vi "Lab Panel V5.22.vi"() -> ()   [LabVIEW 2013] (continued)
                                n836 = local write "DISP LAB03-2"(w1475) -> ()
                              }
                              frame #4 {
                                n837 = local read "TEMP START LAB03-2"() -> (w1494:cluster{"TL":dbl, "TN":dbl})
                                n838 = Bundle(cluster=w1494, "TL"=w1492, "TN"=w1492) -> (w1493:cluster{"TL":dbl, "TN":dbl})
                                n839 = local write "TEMP START LAB03-2"(w1493) -> ()
                              }
                            }
                          }
                        }
                      }
                    }
                  }
                }
              }
              event "RUN LAB04-1": Value Change {
                n840 = event-data() -> ("NewVal"=w1499:bool)  [unwired: 1 in, 5 out]
                n841 = local write "run lab04-1"(w1499) -> ()
                n842 = case shown="True" w1499 {
                  tunnel: w1505 -> [_ w1543]
                  tunnel: w1504 -> [_ w1542]
                  tunnel: w1502 -> [w1507 w1541]
                  tunnel: w1503 -> [_ w1540]
                  tunnel: w1501 -> [_ w1539]
                  tunnel: [w1506 w1538] -> w1500
                  tunnel: w1498 -> [_ w1537]
                  tunnel: w1497 -> [_ w1536]
                  tunnel: w1496 -> [_ w1535]
                  tunnel: w1495 -> [_ w1533]
                  frame False {
                    # "stop test"
                    n843 = stacked-sequence {
                      tunnel: w1507 -> [w1516 _]
                      tunnel: [w1508 _] -> w1506
                      frame #0 {
                        n844 = local read "DISP LAB04-1"() -> (w1515:T4)
                        n845 = Unbundle(w1515) -> ("CYCLE"=w1513:dbl, "MINS"=w1514:dbl)  [unwired: 1 out]
                        n846 = case shown="\"CYCLE TEST\"" w1516 {
                          tunnel: w1514 -> [_ _ w1523]
                          tunnel: w1513 -> [w1521 w1522 _]
                          tunnel: [w1521 w1522 w1523] -> w1512
                          frame "CHART TEST", Default {
                          }
                          frame "CYCLE TEST" {
                          }
                          frame "T-RISE TEST" {
                          }
                        }
                        n847 = local read "TDMS LAB04-1"() -> (w1520:refnum<k34>)
                        n848 = Build Array("STOPPED") -> (w1517:string[])
                        n849 = Build Array(w1512) -> (w1511:dbl[])
                        n850 = TDMS Write(0:w1520, 5:"TEST RESULT", 7:w1517, 9:w1511) -> (4:w1509:refnum<k34>, 15:w1510:errorcluster)  [unwired: 2 in, 2 out]
                        n851 = TDMS Close(8:w1510, 11:w1509) -> (0:w1508:errorcluster)  [unwired: 1 out]
                      }
                      frame #1 {
                        n852 = local read "DISP LAB04-1"() -> (w1527:T4)
                        n853 = stacked-sequence {
                          tunnel: "LAB04-1" -> [w1529 w1531]
                          frame #0 {
                            n854 = call "sub vi - defrag tdms v1.vi"("panel id"=w1529) -> ("error out"=w1528:errorcluster)  [unwired: 10 in]
                            n855 = local write "data file error"(w1528) -> ()
                          }
                          frame #1 {
                            n856 = call "Save data file (stop) v3.vi"("panel id"=w1531) -> ("network file save error"=w1530:errorcluster)  [unwired: 9 in, 1 out]
                            n857 = local write "RESULT LAB04-1"(FALSE) -> ()
                            n858 = local write "data file error"(w1530) -> ()
                          }
                        }
                        n859 = Bundle(cluster=w1527, "STATUS"="STOP") -> (w1525:T4)  [unwired: 2 in]
                        n860 = local write "DISP LAB04-1"(w1525) -> ()
                      }
                    }
                  }
                  frame True {
                    n861 = local read "SIG LAB04-1"() -> (w1534:T2)
                    n862 = stacked-sequence {
                      seq-local: [w1545 _] -> [_ w1549]
                      tunnel: w1543 -> [_ w1559]
                      tunnel: w1542 -> [_ w1558]
                      tunnel: w1541 -> [_ w1557]
                      tunnel: w1540 -> [_ w1556]
                      tunnel: w1539 -> [_ w1555]
                      tunnel: [_ w1554] -> w1538
                      tunnel: w1537 -> [_ w1553]
                      tunnel: w1536 -> [_ w1552]
                      tunnel: w1535 -> [_ w1551]
                      tunnel: w1534 -> [w1544 w1550]
                      tunnel: w1533 -> [_ w1548]
                      frame #0 {
                        n863 = Unbundle(w1544) -> ("AMPS"=w1547:dbl)  [unwired: 4 out]
                        n864 = call "Check For Amps on v1.vi"("ID"="LAB04-1", "amps"=w1547) -> ("amps"=w1545:bool)  [unwired: 9 in]
                      }
                      frame #1 {
                        n865 = case shown="True" w1549 {
                          tunnel: w1559 -> [_ w1572]
                          tunnel: w1558 -> [_ w1571]
                          tunnel: w1557 -> [_ w1570]
                          tunnel: w1556 -> [_ w1569]
                          tunnel: w1555 -> [_ w1568]
                          tunnel: [errorcluster {"status"=FALSE, "code"=0, "source"=""} ("error out") w1567] -> w1554
                          tunnel: w1553 -> [_ w1566]
                          tunnel: w1552 -> [_ w1565]
                          tunnel: w1551 -> [_ w1564]
                          tunnel: w1550 -> [_ w1563]
                          tunnel: w1548 -> [_ w1562]
                          frame False {
                            w1560 = FALSE
                            n866 = local write "RUN LAB04-1"(w1560) -> ()
                            n867 = local write "run lab04-1"(w1560) -> ()
                          }
                          frame True {
                            n868 = stacked-sequence {
                              seq-local: [w1573 _ _ _ _] -> [_ w1597 _ _ _]
                              tunnel: w1572 -> [w1578 _ _ _ _]
                              tunnel: w1571 -> [w1574 _ _ _ _]
                              tunnel: w1570 -> [w1588 _ _ _ _]
                              tunnel: w1569 -> [w1581 _ _ _ _]
                              tunnel: w1568 -> [w1576 _ _ _ _]
                              tunnel: [_ w1592 _ _ _] -> w1567
                              tunnel: w1566 -> [_ _ _ w1618 _]
                              tunnel: w1565 -> [_ _ _ w1617 _]
                              tunnel: w1564 -> [_ _ _ w1616 _]
                              tunnel: w1563 -> [_ _ _ _ _]
                              tunnel: w1562 -> [_ _ _ _ w1632]
                              frame #0 {
                                w1575 = "\\"
                                n869 = local read "SET LAB04-1"() -> (w1583:T5)
                                n870 = case shown="\"CYCLE TEST\"" w1588 {
                                tunnel: ["L04-1-CHART TEST-" "L04-1-CYCLE TEST-" "L04-1-T-RISE TEST-"] -> w1584
                                frame "CHART TEST", Default {
                                }
                                frame "CYCLE TEST" {
                                }
                                frame "T-RISE TEST" {
                                }
                                }
                                n871 = Unbundle(w1583) -> ("DESCRIPTION"=w1582:string)  [unwired: 4 out]
                                n872 = Concatenate Strings(w1578, "\\", w1576, w1575, w1574, w1575) -> (w1585:string)
                                n873 = String To Path(string=w1585) -> (path=w1587:path)
                                n874 = Concatenate Strings(w1585, w1584, w1582, "-", w1581, ".tdms") -> (w1573:string)
                                n875 = Create Folder(path (use dialog)=w1587) -> (error out=w1586:errorcluster)  [unwired: 2 in, 2 out]
                                n876 = global write "Global 1.vi" "LAB04-1 FILE"(w1573) -> ()
                                n877 = call <vilib>:"Clear Errors.vi"("error in (no error)"=w1586) -> ()  [unwired: 6 in, 1 out]
                              }
                              frame #1 {
                                (unwired) FALSE
                                n878 = String To Path(string=w1597) -> (path=w1593:path)
                                n879 = TDMS Open(6:FALSE, 10:T20."create or replace" ("operation (0:open)"), 11:w1593) -> (0:w1592:errorcluster, 3:→"TDMS LAB04-1":refnum<k34>)  [unwired: 4 in]
                              }
                              frame #2 {
                                n880 = local read "SET LAB04-1"() -> (w1603:T5)
                                n881 = local read "TDMS LAB04-1"() -> (w1614:refnum<k34>)
                                n882 = Build Array("Testers Name", "Description", "Set Test Cycles", "T-Rise minutes", "T-Rise Deg C") -> (w1604:string[])
                                n883 = Unbundle(w1603) -> ("NAME"=w1602:string, "DESCRIPTION"=w1601:string, "CYCLES"=w1600:dbl, "T-RISE mins"=w1599:dbl, "T-RISE deg C"=w1598:dbl)
                                n884 = Number To Decimal String(number=w1600) -> (decimal integer string=w1613:string)  [unwired: 1 in]
                                n885 = Number To Decimal String(number=w1599) -> (decimal integer string=w1612:string)  [unwired: 1 in]
                                n886 = Number To Decimal String(number=w1598) -> (decimal integer string=w1611:string)  [unwired: 1 in]
                                n887 = Build Array(w1602, w1601, w1613, w1612, w1611) -> (w1610:string[])
                                n888 = TDMS Set Properties(5:w1610, 7:w1604, 11:w1614) -> ()  [unwired: 3 in, 4 out]
                              }
                              frame #3 {
                                n889 = local read "DISP LAB04-1"() -> (w1619:T4)
                                n890 = Concatenate Strings("LAB04-1  ", w1618) -> (w1620:string)
                                n891 = Two Button Dialog(message=w1620, 1:w1616, 2:w1617) -> (T button?=w1622:bool)
                                n892 = case shown="True" w1622 {
                                tunnel: w1619 -> [w1629 w1630]
                                tunnel: [w1629 w1630] -> w1626
                                tunnel: [w1628 w1631] -> w1625
                                tunnel: [w1627 w1631] -> w1624
                                frame False {
                                n893 = Unbundle(w1629) -> ("CYCLE"=w1628:dbl, "MINS"=w1627:dbl)  [unwired: 1 out]
                                }
                                frame True {
                                w1631 = 0.0
                                }
                                }
                                n894 = Bundle(cluster=w1626, "CYCLE"=w1625, "MINS"=w1624, "STATUS"="RUN") -> (w1615:T4)
                                n895 = local write "DISP LAB04-1"(w1615) -> ()
                              }
                              frame #4 {
                                n896 = local read "TEMP START LAB04-1"() -> (w1634:cluster{"TL":dbl, "TN":dbl})
                                n897 = Bundle(cluster=w1634, "TL"=w1632, "TN"=w1632) -> (w1633:cluster{"TL":dbl, "TN":dbl})
                                n898 = local write "TEMP START LAB04-1"(w1633) -> ()
                              }
                            }
                          }
                        }
                      }
                    }
                  }
                }
              }
              event "RUN LAB04-2": Value Change {
                n899 = event-data() -> ("NewVal"=w1639:bool)  [unwired: 1 in, 5 out]
                n900 = local write "run lab04-2"(w1639) -> ()
                n901 = case shown="True" w1639 {
                  tunnel: w1645 -> [_ w1683]
                  tunnel: w1644 -> [_ w1682]
                  tunnel: w1642 -> [w1647 w1681]
                  tunnel: w1643 -> [_ w1680]
                  tunnel: w1641 -> [_ w1679]
                  tunnel: [w1646 w1678] -> w1640
                  tunnel: w1638 -> [_ w1677]
                  tunnel: w1637 -> [_ w1676]
                  tunnel: w1636 -> [_ w1675]
                  tunnel: w1635 -> [_ w1673]
                  frame False {
                    # "stop test"
                    n902 = stacked-sequence {
                      tunnel: w1647 -> [w1656 _]
                      tunnel: [w1648 _] -> w1646
                      frame #0 {
                        n903 = local read "DISP LAB04-2"() -> (w1655:T4)
                        n904 = Unbundle(w1655) -> ("CYCLE"=w1653:dbl, "MINS"=w1654:dbl)  [unwired: 1 out]
                        n905 = case shown="\"CYCLE TEST\"" w1656 {
                          tunnel: w1654 -> [_ _ w1663]
                          tunnel: w1653 -> [w1661 w1662 _]
                          tunnel: [w1661 w1662 w1663] -> w1652
                          frame "CHART TEST", Default {
                          }
                          frame "CYCLE TEST" {
                          }
                          frame "T-RISE TEST" {
                          }
                        }
                        n906 = local read "TDMS LAB04-2"() -> (w1660:refnum<k34>)
                        n907 = Build Array("STOPPED") -> (w1657:string[])
                        n908 = Build Array(w1652) -> (w1651:dbl[])
                        n909 = TDMS Write(0:w1660, 5:"TEST RESULT", 7:w1657, 9:w1651) -> (4:w1649:refnum<k34>, 15:w1650:errorcluster)  [unwired: 2 in, 2 out]
                        n910 = TDMS Close(8:w1650, 11:w1649) -> (0:w1648:errorcluster)  [unwired: 1 out]
                      }
                      frame #1 {
                        n911 = local read "DISP LAB04-2"() -> (w1667:T4)
                        n912 = stacked-sequence {
                          tunnel: "LAB04-2" -> [w1669 w1671]
                          frame #0 {
                            n913 = call "sub vi - defrag tdms v1.vi"("panel id"=w1669) -> ("error out"=w1668:errorcluster)  [unwired: 10 in]
                            n914 = local write "data file error"(w1668) -> ()
                          }
                          frame #1 {
                            n915 = call "Save data file (stop) v3.vi"("panel id"=w1671) -> ("network file save error"=w1670:errorcluster)  [unwired: 9 in, 1 out]
                            n916 = local write "RESULT LAB04-2"(FALSE) -> ()
                            n917 = local write "data file error"(w1670) -> ()
                          }
                        }
                        n918 = Bundle(cluster=w1667, "STATUS"="STOP") -> (w1665:T4)  [unwired: 2 in]
                        n919 = local write "DISP LAB04-2"(w1665) -> ()
                      }
                    }
                  }
                  frame True {
                    n920 = local read "SIG LAB04-2"() -> (w1674:T2)
                    n921 = stacked-sequence {
                      seq-local: [w1685 _] -> [_ w1689]
                      tunnel: w1683 -> [_ w1699]
                      tunnel: w1682 -> [_ w1698]
                      tunnel: w1681 -> [_ w1697]
                      tunnel: w1680 -> [_ w1696]
                      tunnel: w1679 -> [_ w1695]
                      tunnel: [_ w1694] -> w1678
                      tunnel: w1677 -> [_ w1693]
                      tunnel: w1676 -> [_ w1692]
                      tunnel: w1675 -> [_ w1691]
                      tunnel: w1674 -> [w1684 w1690]
                      tunnel: w1673 -> [_ w1688]
                      frame #0 {
                        n922 = Unbundle(w1684) -> ("AMPS"=w1687:dbl)  [unwired: 4 out]
                        n923 = call "Check For Amps on v1.vi"("ID"="LAB04-2", "amps"=w1687) -> ("amps"=w1685:bool)  [unwired: 9 in]
                      }
                      frame #1 {
                        n924 = case shown="True" w1689 {
                          tunnel: w1699 -> [_ w1712]
                          tunnel: w1698 -> [_ w1711]
                          tunnel: w1697 -> [_ w1710]
                          tunnel: w1696 -> [_ w1709]
                          tunnel: w1695 -> [_ w1708]
                          tunnel: [errorcluster {"status"=FALSE, "code"=0, "source"=""} ("error out") w1707] -> w1694
                          tunnel: w1693 -> [_ w1706]
                          tunnel: w1692 -> [_ w1705]
                          tunnel: w1691 -> [_ w1704]
                          tunnel: w1690 -> [_ w1703]
                          tunnel: w1688 -> [_ w1702]
                          frame False {
                            w1700 = FALSE
                            n925 = local write "RUN LAB04-2"(w1700) -> ()
                            n926 = local write "run lab04-2"(w1700) -> ()
                          }
                          frame True {
                            n927 = stacked-sequence {
                              seq-local: [w1713 _ _ _ _] -> [_ w1737 _ _ _]
                              tunnel: w1712 -> [w1718 _ _ _ _]
                              tunnel: w1711 -> [w1714 _ _ _ _]
                              tunnel: w1710 -> [w1728 _ _ _ _]
                              tunnel: w1709 -> [w1721 _ _ _ _]
                              tunnel: w1708 -> [w1716 _ _ _ _]
                              tunnel: [_ w1732 _ _ _] -> w1707
                              tunnel: w1706 -> [_ _ _ w1758 _]
                              tunnel: w1705 -> [_ _ _ w1757 _]
                              tunnel: w1704 -> [_ _ _ w1756 _]
                              tunnel: w1703 -> [_ _ _ _ _]
                              tunnel: w1702 -> [_ _ _ _ w1772]
                              frame #0 {
                                w1715 = "\\"
                                n928 = local read "SET LAB04-2"() -> (w1723:T5)
                                n929 = case shown="\"CHART TEST\", Default" w1728 {
                                tunnel: ["L04-2-CHART TEST-" "L04-2-CYCLE TEST-" "L04-2-T-RISE TEST-"] -> w1724
                                frame "CHART TEST", Default {
                                }
                                frame "CYCLE TEST" {
                                }
                                frame "T-RISE TEST" {
                                }
                                }
                                n930 = Unbundle(w1723) -> ("DESCRIPTION"=w1722:string)  [unwired: 4 out]
                                n931 = Concatenate Strings(w1718, "\\", w1716, w1715, w1714, w1715) -> (w1725:string)
                                n932 = String To Path(string=w1725) -> (path=w1727:path)
                                n933 = Concatenate Strings(w1725, w1724, w1722, "-", w1721, ".tdms") -> (w1713:string)
                                n934 = Create Folder(path (use dialog)=w1727) -> (error out=w1726:errorcluster)  [unwired: 2 in, 2 out]
                                n935 = global write "Global 1.vi" "LAB04-2 FILE"(w1713) -> ()
                                n936 = call <vilib>:"Clear Errors.vi"("error in (no error)"=w1726) -> ()  [unwired: 6 in, 1 out]
                              }
                              frame #1 {
                                (unwired) FALSE
                                n937 = String To Path(string=w1737) -> (path=w1733:path)
                                n938 = TDMS Open(6:FALSE, 10:T20."create or replace" ("operation (0:open)"), 11:w1733) -> (0:w1732:errorcluster, 3:→"TDMS LAB04-2":refnum<k34>)  [unwired: 4 in]
                              }
                              frame #2 {
                                n939 = local read "SET LAB04-2"() -> (w1743:T5)
                                n940 = local read "TDMS LAB04-2"() -> (w1754:refnum<k34>)
                                n941 = Build Array("Testers Name", "Description", "Set Test Cycles", "T-Rise minutes", "T-Rise Deg C") -> (w1744:string[])
                                n942 = Unbundle(w1743) -> ("NAME"=w1742:string, "DESCRIPTION"=w1741:string, "CYCLES"=w1740:dbl, "T-RISE mins"=w1739:dbl, "T-RISE deg C"=w1738:dbl)
                                n943 = Number To Decimal String(number=w1740) -> (decimal integer string=w1753:string)  [unwired: 1 in]
                                n944 = Number To Decimal String(number=w1739) -> (decimal integer string=w1752:string)  [unwired: 1 in]
                                n945 = Number To Decimal String(number=w1738) -> (decimal integer string=w1751:string)  [unwired: 1 in]
                                n946 = Build Array(w1742, w1741, w1753, w1752, w1751) -> (w1750:string[])
                                n947 = TDMS Set Properties(5:w1750, 7:w1744, 11:w1754) -> ()  [unwired: 3 in, 4 out]
                              }
                              frame #3 {
                                n948 = local read "DISP LAB04-2"() -> (w1759:T4)
                                n949 = Concatenate Strings("LAB04-2 ", w1758) -> (w1760:string)
                                n950 = Two Button Dialog(message=w1760, 1:w1756, 2:w1757) -> (T button?=w1762:bool)
                                n951 = case shown="True" w1762 {
                                tunnel: w1759 -> [w1769 w1770]
                                tunnel: [w1769 w1770] -> w1766
                                tunnel: [w1768 w1771] -> w1765
                                tunnel: [w1767 w1771] -> w1764
                                frame False {
                                n952 = Unbundle(w1769) -> ("CYCLE"=w1768:dbl, "MINS"=w1767:dbl)  [unwired: 1 out]
                                }
                                frame True {
                                w1771 = 0.0
                                }
                                }
                                n953 = Bundle(cluster=w1766, "CYCLE"=w1765, "MINS"=w1764, "STATUS"="RUN") -> (w1755:T4)
                                n954 = local write "DISP LAB04-2"(w1755) -> ()
                              }
                              frame #4 {
                                n955 = local read "TEMP START LAB04-2"() -> (w1774:cluster{"TL":dbl, "TN":dbl})
                                n956 = Bundle(cluster=w1774, "TL"=w1772, "TN"=w1772) -> (w1773:cluster{"TL":dbl, "TN":dbl})
                                n957 = local write "TEMP START LAB04-2"(w1773) -> ()
                              }
                            }
                          }
                        }
                      }
                    }
                  }
                }
              }
              event "RUN LAB05-1": Value Change {
                n958 = event-data() -> ("NewVal"=w1779:bool)  [unwired: 1 in, 5 out]
                n959 = local write "run lab05-1"(w1779) -> ()
                n960 = case shown="True" w1779 {
                  tunnel: w1785 -> [_ w1823]
                  tunnel: w1784 -> [_ w1822]
                  tunnel: w1782 -> [w1787 w1821]
                  tunnel: w1783 -> [_ w1820]
                  tunnel: w1781 -> [_ w1819]
                  tunnel: [w1786 w1818] -> w1780
                  tunnel: w1778 -> [_ w1817]
                  tunnel: w1777 -> [_ w1816]
                  tunnel: w1776 -> [_ w1815]
                  tunnel: w1775 -> [_ w1813]
                  frame False {
                    # "stop test"
                    n961 = stacked-sequence {
                      tunnel: w1787 -> [w1796 _]
                      tunnel: [w1788 _] -> w1786
                      frame #0 {
                        n962 = local read "DISP LAB05-1"() -> (w1795:T4)
                        n963 = Unbundle(w1795) -> ("CYCLE"=w1793:dbl, "MINS"=w1794:dbl)  [unwired: 1 out]
                        n964 = case shown="\"CYCLE TEST\"" w1796 {
                          tunnel: w1794 -> [_ _ w1803]
                          tunnel: w1793 -> [w1801 w1802 _]
                          tunnel: [w1801 w1802 w1803] -> w1792
                          frame "CHART TEST", Default {
                          }
                          frame "CYCLE TEST" {
                          }
                          frame "T-RISE TEST" {
                          }
                        }
                        n965 = local read "TDMS LAB05-1"() -> (w1800:refnum<k34>)
                        n966 = Build Array("STOPPED") -> (w1797:string[])
                        n967 = Build Array(w1792) -> (w1791:dbl[])
                        n968 = TDMS Write(0:w1800, 5:"TEST RESULT", 7:w1797, 9:w1791) -> (4:w1789:refnum<k34>, 15:w1790:errorcluster)  [unwired: 2 in, 2 out]
                        n969 = TDMS Close(8:w1790, 11:w1789) -> (0:w1788:errorcluster)  [unwired: 1 out]
                      }
                      frame #1 {
                        n970 = local read "DISP LAB05-1"() -> (w1807:T4)
                        n971 = stacked-sequence {
                          tunnel: "LAB05-1" -> [w1809 w1811]
                          frame #0 {
                            n972 = call "sub vi - defrag tdms v1.vi"("panel id"=w1809) -> ("error out"=w1808:errorcluster)  [unwired: 10 in]
                            n973 = local write "data file error"(w1808) -> ()
                          }
                          frame #1 {
                            n974 = call "Save data file (stop) v3.vi"("panel id"=w1811) -> ("network file save error"=w1810:errorcluster)  [unwired: 9 in, 1 out]
                            n975 = local write "RESULT LAB05-1"(FALSE) -> ()
                            n976 = local write "data file error"(w1810) -> ()
                          }
                        }
                        n977 = Bundle(cluster=w1807, "STATUS"="STOP") -> (w1805:T4)  [unwired: 2 in]
                        n978 = local write "DISP LAB05-1"(w1805) -> ()
                      }
                    }
                  }
                  frame True {
                    n979 = local read "SIG LAB05-1"() -> (w1814:T2)
                    n980 = stacked-sequence {
                      seq-local: [w1825 _] -> [_ w1829]
                      tunnel: w1823 -> [_ w1839]
                      tunnel: w1822 -> [_ w1838]
                      tunnel: w1821 -> [_ w1837]
                      tunnel: w1820 -> [_ w1836]
                      tunnel: w1819 -> [_ w1835]
                      tunnel: [_ w1834] -> w1818
                      tunnel: w1817 -> [_ w1833]
                      tunnel: w1816 -> [_ w1832]
                      tunnel: w1815 -> [_ w1831]
                      tunnel: w1814 -> [w1824 w1830]
                      tunnel: w1813 -> [_ w1828]
                      frame #0 {
                        n981 = Unbundle(w1824) -> ("AMPS"=w1827:dbl)  [unwired: 4 out]
                        n982 = call "Check For Amps on v1.vi"("ID"="LAB05-1", "amps"=w1827) -> ("amps"=w1825:bool)  [unwired: 9 in]
                      }
                      frame #1 {
                        n983 = case shown="True" w1829 {
                          tunnel: w1839 -> [_ w1852]
                          tunnel: w1838 -> [_ w1851]
                          tunnel: w1837 -> [_ w1850]
                          tunnel: w1836 -> [_ w1849]
                          tunnel: w1835 -> [_ w1848]
                          tunnel: [errorcluster {"status"=FALSE, "code"=0, "source"=""} ("error out") w1847] -> w1834
                          tunnel: w1833 -> [_ w1846]
                          tunnel: w1832 -> [_ w1845]
                          tunnel: w1831 -> [_ w1844]
                          tunnel: w1830 -> [_ w1843]
                          tunnel: w1828 -> [_ w1842]
                          frame False {
                            w1840 = FALSE
                            n984 = local write "RUN LAB05-1"(w1840) -> ()
                            n985 = local write "run lab05-1"(w1840) -> ()
                          }
                          frame True {
                            n986 = stacked-sequence {
                              seq-local: [w1853 _ _ _ _] -> [_ w1877 _ _ _]
                              tunnel: w1852 -> [w1858 _ _ _ _]
                              tunnel: w1851 -> [w1854 _ _ _ _]
                              tunnel: w1850 -> [w1868 _ _ _ _]
                              tunnel: w1849 -> [w1861 _ _ _ _]
                              tunnel: w1848 -> [w1856 _ _ _ _]
                              tunnel: [_ w1872 _ _ _] -> w1847
                              tunnel: w1846 -> [_ _ _ w1897 _]
                              tunnel: w1845 -> [_ _ _ w1896 _]
                              tunnel: w1844 -> [_ _ _ w1895 _]
                              tunnel: w1843 -> [_ _ _ _ _]
                              tunnel: w1842 -> [_ _ _ _ w1912]
                              frame #0 {
                                w1855 = "\\"
                                n987 = local read "SET LAB05-1"() -> (w1863:T5)
                                n988 = case shown="\"CYCLE TEST\"" w1868 {
                                tunnel: ["L05-1-CHART TEST-" "L05-1-CYCLE TEST-" "L05-1-T-RISE TEST-"] -> w1864
                                frame "CHART TEST", Default {
                                }
                                frame "CYCLE TEST" {
                                }
                                frame "T-RISE TEST" {
                                }
                                }
                                n989 = Unbundle(w1863) -> ("DESCRIPTION"=w1862:string)  [unwired: 4 out]
                                n990 = Concatenate Strings(w1858, "\\", w1856, w1855, w1854, w1855) -> (w1865:string)
                                n991 = String To Path(string=w1865) -> (path=w1867:path)
                                n992 = Concatenate Strings(w1865, w1864, w1862, "-", w1861, ".tdms") -> (w1853:string)
                                n993 = Create Folder(path (use dialog)=w1867) -> (error out=w1866:errorcluster)  [unwired: 2 in, 2 out]
                                n994 = global write "Global 1.vi" "LAB05-1 FILE"(w1853) -> ()
                                n995 = call <vilib>:"Clear Errors.vi"("error in (no error)"=w1866) -> ()  [unwired: 6 in, 1 out]
                              }
                              frame #1 {
                                (unwired) FALSE
                                n996 = String To Path(string=w1877) -> (path=w1873:path)
                                n997 = TDMS Open(6:FALSE, 10:T20."create or replace" ("operation (0:open)"), 11:w1873) -> (0:w1872:errorcluster, 3:→"TDMS LAB05-1":refnum<k34>)  [unwired: 4 in]
                              }
                              frame #2 {
                                n998 = local read "SET LAB05-1"() -> (w1883:T5)
                                n999 = local read "TDMS LAB05-1"() -> (w1894:refnum<k34>)
                                n1000 = Build Array("Testers Name", "Description", "Set Test Cycles", "T-Rise minutes", "T-Rise Deg C") -> (w1884:string[])
                                n1001 = Unbundle(w1883) -> ("NAME"=w1882:string, "DESCRIPTION"=w1881:string, "CYCLES"=w1880:dbl, "T-RISE mins"=w1879:dbl, "T-RISE deg C"=w1878:dbl)
                                n1002 = Number To Decimal String(number=w1880) -> (decimal integer string=w1893:string)  [unwired: 1 in]
                                n1003 = Number To Decimal String(number=w1879) -> (decimal integer string=w1892:string)  [unwired: 1 in]
                                n1004 = Number To Decimal String(number=w1878) -> (decimal integer string=w1891:string)  [unwired: 1 in]
                                n1005 = Build Array(w1882, w1881, w1893, w1892, w1891) -> (w1890:string[])
                                n1006 = TDMS Set Properties(5:w1890, 7:w1884, 11:w1894) -> ()  [unwired: 3 in, 4 out]
                              }
                              frame #3 {
                                n1007 = local read "DISP LAB05-1"() -> (w1899:T4)
                                n1008 = Concatenate Strings("LAB05-1  ", w1897) -> (w1900:string)
                                n1009 = Two Button Dialog(message=w1900, 1:w1895, 2:w1896) -> (T button?=w1902:bool)
                                n1010 = case shown="True" w1902 {
                                tunnel: w1899 -> [w1909 w1910]
                                tunnel: [w1909 w1910] -> w1906
                                tunnel: [w1908 w1911] -> w1905
                                tunnel: [w1907 w1911] -> w1904
                                frame False {
                                n1011 = Unbundle(w1909) -> ("CYCLE"=w1908:dbl, "MINS"=w1907:dbl)  [unwired: 1 out]
                                }
                                frame True {
                                w1911 = 0.0
                                }
                                }
                                n1012 = Bundle(cluster=w1906, "CYCLE"=w1905, "MINS"=w1904, "STATUS"="RUN") -> (w1898:T4)
                                n1013 = local write "DISP LAB05-1"(w1898) -> ()
                              }
                              frame #4 {
                                n1014 = local read "TEMP START LAB05-1"() -> (w1914:cluster{"TL":dbl, "TN":dbl})
                                n1015 = Bundle(cluster=w1914, "TL"=w1912, "TN"=w1912) -> (w1913:cluster{"TL":dbl, "TN":dbl})
                                n1016 = local write "TEMP START LAB05-1"(w1913) -> ()
                              }
                            }
                          }
                        }
                      }
                    }
                  }
                }
              }
              event "RUN LAB05-2": Value Change {
                n1017 = event-data() -> ("NewVal"=w1920:bool)  [unwired: 1 in, 5 out]
                n1018 = local read "SIG LAB05-2"() -> (w1916:T2)
                n1019 = case shown="True" w1920 {
                  tunnel: w1926 -> [_ w1964]
                  tunnel: w1925 -> [_ w1963]
                  tunnel: w1923 -> [w1928 w1962]
                  tunnel: w1924 -> [_ w1961]
                  tunnel: w1922 -> [_ w1960]
                  tunnel: [w1927 w1959] -> w1921
                  tunnel: w1919 -> [_ w1958]
                  tunnel: w1918 -> [_ w1957]
                  tunnel: w1917 -> [_ w1956]
                  tunnel: w1916 -> [_ w1955]
                  tunnel: w1915 -> [_ w1954]
                  frame False {
                    # "stop test"
                    n1020 = stacked-sequence {
                      tunnel: w1928 -> [w1937 _]
                      tunnel: [w1929 _] -> w1927
                      frame #0 {
                        n1021 = local read "DISP LAB05-2"() -> (w1936:T4)
                        n1022 = Unbundle(w1936) -> ("CYCLE"=w1934:dbl, "MINS"=w1935:dbl)  [unwired: 1 out]
                        n1023 = case shown="\"CYCLE TEST\"" w1937 {
                          tunnel: w1935 -> [_ _ w1944]
                          tunnel: w1934 -> [w1942 w1943 _]
                          tunnel: [w1942 w1943 w1944] -> w1933
                          frame "CHART TEST", Default {
                          }
                          frame "CYCLE TEST" {
                          }
                          frame "T-RISE TEST" {
                          }
                        }
                        n1024 = local read "TDMS LAB05-2"() -> (w1941:refnum<k34>)
                        n1025 = Build Array("STOPPED") -> (w1938:string[])
                        n1026 = Build Array(w1933) -> (w1932:dbl[])
                        n1027 = TDMS Write(0:w1941, 5:"TEST RESULT", 7:w1938, 9:w1932) -> (4:w1930:refnum<k34>, 15:w1931:errorcluster)  [unwired: 2 in, 2 out]
                        n1028 = TDMS Close(8:w1931, 11:w1930) -> (0:w1929:errorcluster)  [unwired: 1 out]
                      }
                      frame #1 {
                        n1029 = local read "DISP LAB05-2"() -> (w1948:T4)
                        n1030 = stacked-sequence {
                          tunnel: "LAB05-2" -> [w1950 w1952]
                          frame #0 {
                            n1031 = call "sub vi - defrag tdms v1.vi"("panel id"=w1950) -> ("error out"=w1949:errorcluster)  [unwired: 10 in]
                            n1032 = local write "data file error"(w1949) -> ()
                          }
                          frame #1 {
                            n1033 = local write "RESULT LAB05-2"(FALSE) -> ()
                            n1034 = call "Save data file (stop) v3.vi"("panel id"=w1952) -> ("network file save error"=w1951:errorcluster)  [unwired: 9 in, 1 out]
                            n1035 = local write "data file error"(w1951) -> ()
                          }
                        }
                        n1036 = Bundle(cluster=w1948, "STATUS"="STOP") -> (w1946:T4)  [unwired: 2 in]
                        n1037 = local write "DISP LAB05-2"(w1946) -> ()
                      }
                    }
                  }
                  frame True {
                    n1038 = stacked-sequence {
                      seq-local: [w1966 _] -> [_ w1970]
                      tunnel: w1964 -> [_ w1980]
                      tunnel: w1963 -> [_ w1979]
                      tunnel: w1962 -> [_ w1978]
                      tunnel: w1961 -> [_ w1977]
                      tunnel: w1960 -> [_ w1976]
                      tunnel: [_ w1975] -> w1959
                      tunnel: w1958 -> [_ w1974]
                      tunnel: w1957 -> [_ w1973]
                      tunnel: w1956 -> [_ w1972]
                      tunnel: w1955 -> [w1965 w1971]
                      tunnel: w1954 -> [_ w1969]
                      frame #0 {
                        n1039 = Unbundle(w1965) -> ("AMPS"=w1968:dbl)  [unwired: 4 out]
                        n1040 = call "Check For Amps on v1.vi"("ID"="LAB05-2", "amps"=w1968) -> ("amps"=w1966:bool)  [unwired: 9 in]
                      }
                      frame #1 {
                        n1041 = case shown="True" w1970 {
                          tunnel: w1980 -> [_ w1993]
                          tunnel: w1979 -> [_ w1992]
                          tunnel: w1978 -> [_ w1991]
                          tunnel: w1977 -> [_ w1990]
                          tunnel: w1976 -> [_ w1989]
                          tunnel: [errorcluster {"status"=FALSE, "code"=0, "source"=""} ("error out") w1988] -> w1975
                          tunnel: w1974 -> [_ w1987]
                          tunnel: w1973 -> [_ w1986]
                          tunnel: w1972 -> [_ w1985]
                          tunnel: w1971 -> [_ w1984]
                          tunnel: w1969 -> [_ w1983]
                          frame False {
                            w1981 = FALSE
                            n1042 = local write "RUN LAB05-2"(w1981) -> ()
                            n1043 = local write "run lab05-2"(w1981) -> ()
                          }
                          frame True {
                            n1044 = stacked-sequence {
                              seq-local: [w1994 _ _ _ _] -> [_ w2018 _ _ _]
                              tunnel: w1993 -> [w1999 _ _ _ _]
                              tunnel: w1992 -> [w1995 _ _ _ _]
                              tunnel: w1991 -> [w2009 _ _ _ _]
                              tunnel: w1990 -> [w2002 _ _ _ _]
                              tunnel: w1989 -> [w1997 _ _ _ _]
                              tunnel: [_ w2013 _ _ _] -> w1988
                              tunnel: w1987 -> [_ _ _ w2038 _]
                              tunnel: w1986 -> [_ _ _ w2037 _]
                              tunnel: w1985 -> [_ _ _ w2036 _]
                              tunnel: w1984 -> [_ _ _ _ _]
                              tunnel: w1983 -> [_ _ _ _ w2053]
                              frame #0 {
                                w1996 = "\\"
                                n1045 = local read "SET LAB05-2"() -> (w2004:T5)
                                n1046 = case shown="\"CYCLE TEST\"" w2009 {
                                tunnel: ["L05-2-CHART TEST-" "L05-2-CYCLE TEST-" "L05-2-T-RISE TEST-"] -> w2005
                                frame "CHART TEST", Default {
                                }
                                frame "CYCLE TEST" {
                                }
                                frame "T-RISE TEST" {
                                }
                                }
                                n1047 = Unbundle(w2004) -> ("DESCRIPTION"=w2003:string)  [unwired: 4 out]
                                n1048 = Concatenate Strings(w1999, "\\", w1997, w1996, w1995, w1996) -> (w2006:string)
                                n1049 = String To Path(string=w2006) -> (path=w2008:path)
                                n1050 = Concatenate Strings(w2006, w2005, w2003, "-", w2002, ".tdms") -> (w1994:string)
                                n1051 = Create Folder(path (use dialog)=w2008) -> (error out=w2007:errorcluster)  [unwired: 2 in, 2 out]
                                n1052 = global write "Global 1.vi" "LAB05-2 FILE"(w1994) -> ()
                                n1053 = call <vilib>:"Clear Errors.vi"("error in (no error)"=w2007) -> ()  [unwired: 6 in, 1 out]
                              }
                              frame #1 {
                                (unwired) FALSE
                                n1054 = String To Path(string=w2018) -> (path=w2014:path)
                                n1055 = TDMS Open(6:FALSE, 10:T20."create or replace" ("operation (0:open)"), 11:w2014) -> (0:w2013:errorcluster, 3:→"TDMS LAB05-2":refnum<k34>)  [unwired: 4 in]
                              }
                              frame #2 {
                                n1056 = local read "SET LAB05-2"() -> (w2024:T5)
                                n1057 = local read "TDMS LAB05-2"() -> (w2035:refnum<k34>)
                                n1058 = Build Array("Testers Name", "Description", "Set Test Cycles", "T-Rise minutes", "T-Rise Deg C") -> (w2025:string[])
                                n1059 = Unbundle(w2024) -> ("NAME"=w2023:string, "DESCRIPTION"=w2022:string, "CYCLES"=w2021:dbl, "T-RISE mins"=w2020:dbl, "T-RISE deg C"=w2019:dbl)
                                n1060 = Number To Decimal String(number=w2021) -> (decimal integer string=w2034:string)  [unwired: 1 in]
                                n1061 = Number To Decimal String(number=w2020) -> (decimal integer string=w2033:string)  [unwired: 1 in]
                                n1062 = Number To Decimal String(number=w2019) -> (decimal integer string=w2032:string)  [unwired: 1 in]
                                n1063 = Build Array(w2023, w2022, w2034, w2033, w2032) -> (w2031:string[])
                                n1064 = TDMS Set Properties(5:w2031, 7:w2025, 11:w2035) -> ()  [unwired: 3 in, 4 out]
                              }
                              frame #3 {
                                n1065 = local read "DISP LAB05-2"() -> (w2040:T4)
                                n1066 = Concatenate Strings("LAB05-2  ", w2038) -> (w2041:string)
                                n1067 = Two Button Dialog(message=w2041, 1:w2036, 2:w2037) -> (T button?=w2043:bool)
                                n1068 = case shown="True" w2043 {
                                tunnel: w2040 -> [w2050 w2051]
                                tunnel: [w2050 w2051] -> w2047
                                tunnel: [w2049 w2052] -> w2046
                                tunnel: [w2048 w2052] -> w2045
                                frame False {
                                n1069 = Unbundle(w2050) -> ("CYCLE"=w2049:dbl, "MINS"=w2048:dbl)  [unwired: 1 out]
                                }
                                frame True {
                                w2052 = 0.0
                                }
                                }
                                n1070 = Bundle(cluster=w2047, "CYCLE"=w2046, "MINS"=w2045, "STATUS"="RUN") -> (w2039:T4)
                                n1071 = local write "DISP LAB05-2"(w2039) -> ()
                              }
                              frame #4 {
                                n1072 = local read "TEMP START LAB05-2"() -> (w2055:cluster{"TL":dbl, "TN":dbl})
                                n1073 = Bundle(cluster=w2055, "TL"=w2053, "TN"=w2053) -> (w2054:cluster{"TL":dbl, "TN":dbl})
                                n1074 = local write "TEMP START LAB05-2"(w2054) -> ()
                              }
                            }
                          }
                        }
                      }
                    }
                  }
                }
                n1075 = local write "run lab05-2"(w1920) -> ()
              }
            }
            n1076 = local write "data file error"(w624) -> ()
          }
          frame #4 {
            # "check if test cycles reached for cycle tests, if so then test pass"
            n1077 = stacked-sequence {
              tunnel: w2075 -> [_ _ _ _ _ _ _ _ _ _]
              tunnel: w2074 -> [_ _ _ _ _ _ _ _ _ _]
              tunnel: w2073 -> [_ _ _ _ _ _ _ _ _ _]
              tunnel: w2072 -> [_ _ _ _ _ _ _ _ _ _]
              tunnel: w2071 -> [_ _ _ _ _ _ _ _ _ _]
              tunnel: w2070 -> [_ _ _ _ _ _ _ _ _ _]
              tunnel: w2069 -> [_ _ _ _ _ _ _ _ _ _]
              tunnel: w2068 -> [_ _ _ _ _ _ _ _ _ _]
              tunnel: w2067 -> [_ _ _ _ _ _ _ _ _ _]
              tunnel: w2066 -> [_ _ _ _ _ _ _ _ _ _]
              tunnel: w2065 -> [w2081 _ _ _ _ _ _ _ _ _]
              tunnel: w2064 -> [_ w2116 _ _ _ _ _ _ _ _]
              tunnel: w2063 -> [_ _ w2156 _ _ _ _ _ _ _]
              tunnel: w2062 -> [_ _ _ w2196 _ _ _ _ _ _]
              tunnel: w2061 -> [_ _ _ _ w2236 _ _ _ _ _]
              tunnel: w2060 -> [_ _ _ _ _ w2276 _ _ _ _]
              tunnel: w2059 -> [_ _ _ _ _ _ w2316 _ _ _]
              tunnel: w2058 -> [_ _ _ _ _ _ _ w2356 _ _]
              tunnel: w2057 -> [_ _ _ _ _ _ _ _ w2396 _]
              tunnel: w2056 -> [_ _ _ _ _ _ _ _ _ w2436]
              frame #0 {
                # "LAB01-1"
                n1078 = Less?(x=w2081, y=2) -> (x < y?=w2079:bool)
                n1079 = local read "DISP LAB01-1"() -> (w2082:T4)
                n1080 = Unbundle(w2082) -> ("STATUS"=w2076:string)  [unwired: 2 out]
                n1081 = Equal?(x=w2076, y="RUN") -> (x = y?=w2078:bool)
                n1082 = And(x=w2078, y=w2079) -> (x .and. y?=w2077:bool)
                n1083 = case shown="True" w2077 {
                  tunnel: w2082 -> [_ w2087]
                  tunnel: w2081 -> [_ w2091]
                  frame False {
                  }
                  frame True {
                    n1084 = local read "SET LAB01-1"() -> (w2093:T5)
                    n1085 = local read "TDMS LAB01-1"() -> (w2086:refnum<k34>)
                    n1086 = Unbundle(w2093) -> ("CYCLES"=w2084:dbl, "T-RISE mins"=w2090:dbl)  [unwired: 3 out]
                    n1087 = case shown="\"CYCLE TEST\"" w2091 {
                      tunnel: w2090 -> [_ _ w2100]
                      tunnel: [w2095 w2097 w2100] -> w2089
                      tunnel: w2084 -> [w2095 w2097 _]
                      tunnel: ["CHART PASS" "CYCLE PASS" "T-RISE PASS"] -> w2088
                      frame "CHART TEST", Default {
                      }
                      frame "CYCLE TEST" {
                      }
                      frame "T-RISE TEST" {
                      }
                    }
                    n1088 = Unbundle(w2087) -> ("CYCLE"=w2092:dbl)  [unwired: 2 out]
                    n1089 = Increment(x=w2084) -> (x+1=w2085:dbl)
                    n1090 = Greater Or Equal?(x=w2092, y=w2085) -> (x >= y?=w2094:bool)
                    n1091 = case shown="True" w2094 {
                      tunnel: w2089 -> [w2104 _]
                      tunnel: w2088 -> [w2103 _]
                      tunnel: w2087 -> [w2102 _]
                      tunnel: w2086 -> [w2101 _]
                      frame True {
                        n1092 = stacked-sequence {
                          tunnel: w2104 -> [w2108 _]
                          tunnel: w2103 -> [w2106 w2112]
                          tunnel: w2102 -> [_ w2115]
                          tunnel: w2101 -> [w2105 _]
                          frame #0 {
                            n1093 = Build Array(w2106) -> (w2109:string[])
                            n1094 = Build Array(w2108) -> (w2107:dbl[])
                            n1095 = TDMS Write(0:w2105, 5:"TEST PASS", 7:w2109, 9:w2107) -> (15:w2111:errorcluster)  [unwired: 2 in, 3 out]
                            n1096 = local write "data file error"(w2111) -> ()
                          }
                          frame #1 {
                            n1097 = Bundle(cluster=w2115, "STATUS"=w2112) -> (w2113:T4)  [unwired: 2 in]
                            n1098 = local write "RESULT LAB01-1"(TRUE) -> ()
                            n1099 = local write "DISP LAB01-1"(w2113) -> ()
                          }
                        }
                      }
                      frame False {
                      }
                    }
                  }
                }
              }
              frame #1 {
                # "LAB01-2"
                n1100 = Less?(x=w2116, y=2) -> (x < y?=w2119:bool)
                n1101 = local read "DISP LAB01-2"() -> (w2121:T4)
                n1102 = Unbundle(w2121) -> ("STATUS"=w2122:string)  [unwired: 2 out]
                n1103 = Equal?(x=w2122, y="RUN") -> (x = y?=w2118:bool)
                n1104 = And(x=w2118, y=w2119) -> (x .and. y?=w2117:bool)
                n1105 = case shown="True" w2117 {
                  tunnel: w2121 -> [_ w2127]
                  tunnel: w2116 -> [_ w2131]
                  frame False {
                  }
                  frame True {
                    n1106 = local read "SET LAB01-2"() -> (w2133:T5)
                    n1107 = local read "TDMS LAB01-2"() -> (w2126:refnum<k34>)
                    n1108 = Unbundle(w2133) -> ("CYCLES"=w2124:dbl, "T-RISE mins"=w2130:dbl)  [unwired: 3 out]
                    n1109 = case shown="\"T-RISE TEST\"" w2131 {
